vi "Initialize Device Data.vi"(5 "Dropbox Directory":string) -> (1 "GPS Longitude Error":dbl=-121.823962, 2 "GPS Latitude Error":dbl=39.689399, 3 "XBox Device Index":i32)   [LabVIEW 2011]
uses:
  <vilib>/Utility/file.llb/Read From Spreadsheet File (DBL).vi
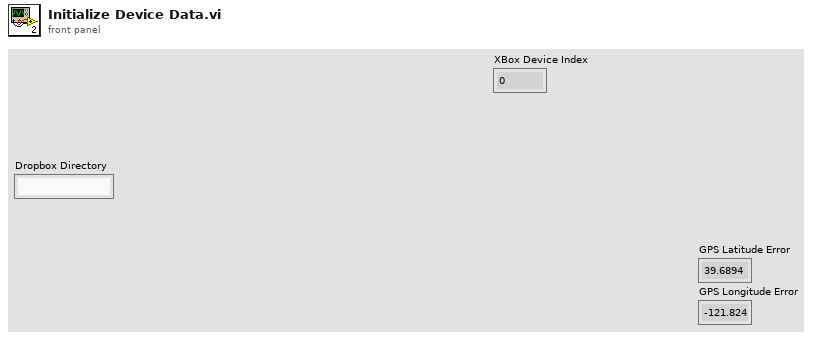
[diagram p1: front panel]
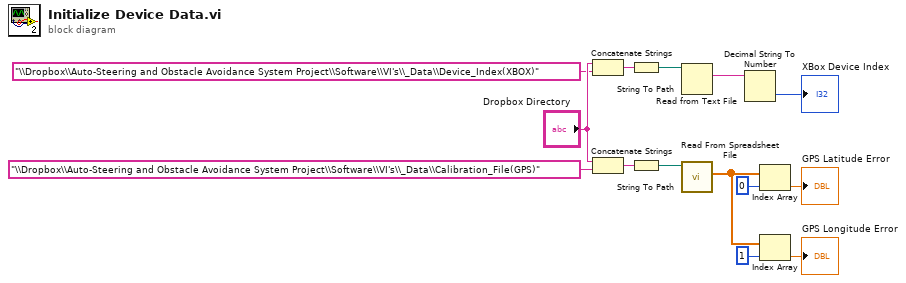
[diagram p0: block diagram]
diagram:
  n1 = Concatenate Strings("Dropbox Directory", "\\Dropbox\\Auto-Steering and Obstacle Avoidance System Project\\Software\\VI's\\_Data\\Device_Index(XBOX)" ("string")) -> (w9:string)
  n2 = Concatenate Strings("Dropbox Directory", "\\Dropbox\\Auto-Steering and Obstacle Avoidance System Project\\Software\\VI's\\_Data\\Calibration_File(GPS)" ("string")) -> (w6:string)
  n3 = String To Path(string=w9) -> (path=w11:path)
  n4 = String To Path(string=w6) -> (path=w8:path)
  n5 = Read from Text File(file (use dialog)=w11) -> (text=w12:string)  [unwired: 3 in, 3 out]
  n6 = call-poly <vilib>:"Read From Spreadsheet File.vi"("file path (dialog if empty)"=w8) -> ("first row"=w3:dbl[])  [unwired: 6 in, 4 out]
  n7 = Decimal String To Number(string=w12) -> (number=→"XBox Device Index":i32)  [unwired: 2 in, 1 out]
  n8 = Index Array(array=w3, index=0) -> (element=→"GPS Latitude Error":dbl)
  n9 = Index Array(array=w3, index=1) -> (element=→"GPS Longitude Error":dbl)
